vi "Subtract.vi"(6 "Z":dbl, 8 "error in (no error)":errorcluster, 9 "Y":dbl, 10 "X":dbl, 11 "Vec3d in":refnum<class "Vec3d.lvclass">) -> (0 "error out":errorcluster, 3 "Vec3d  out":refnum<class "Vec3d.lvclass">)   [LabVIEW 2017, in "Vec3d.lvclass"]
uses:
  Vec3d.lvclass
  Vec3d.lvclass/Vec3d.ctl
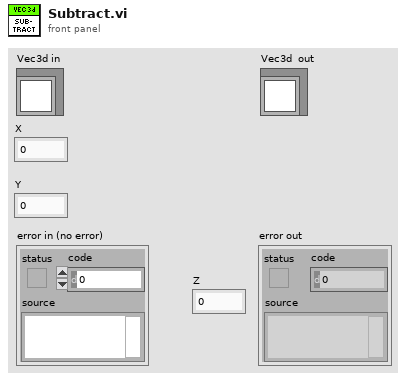
[diagram p1: front panel]
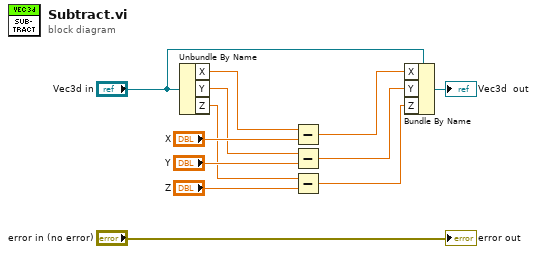
[diagram p0: block diagram]
diagram:
  n1 = Unbundle By Name("Vec3d in") -> ("X"=w9:dbl, "Y"=w8:dbl, "Z"=w7:dbl)
  n2 = Subtract(x=w9, y="X") -> (x-y=w6:dbl)
  n3 = Subtract(x=w8, y="Y") -> (x-y=w5:dbl)
  n4 = Subtract(x=w7, y="Z") -> (x-y=w4:dbl)
  n5 = Bundle By Name(cluster="Vec3d in", "X"=w6, "Y"=w5, "Z"=w4) -> (→"Vec3d  out":refnum<class "Vec3d.lvclass">)
  "error out" <- "error in (no error)"
